vi "Smart_Oscilloscope.vi"() -> ()   [LabVIEW 2024]
uses:
  <vilib>/httpClient/POSTBuffer.vi
  <vilib>/httpClient/LabVIEWHTTPClient.lvlib
panel:
  in  "AI诊断":bool
  out "String":string
  in  "保存数据":bool
  in  "单次采集":bool
  in  "停止程序":bool
  in  "开始采集":bool
  in  "水平基准":dbl(knob) scale=0.0..10.0
  in  "垂直档位":dbl(knob) scale=0.0..10.0
  in  "采样率":dbl(knob) scale=0.0..10.0
  out "Waveform Graph":dynamicdata(graph)
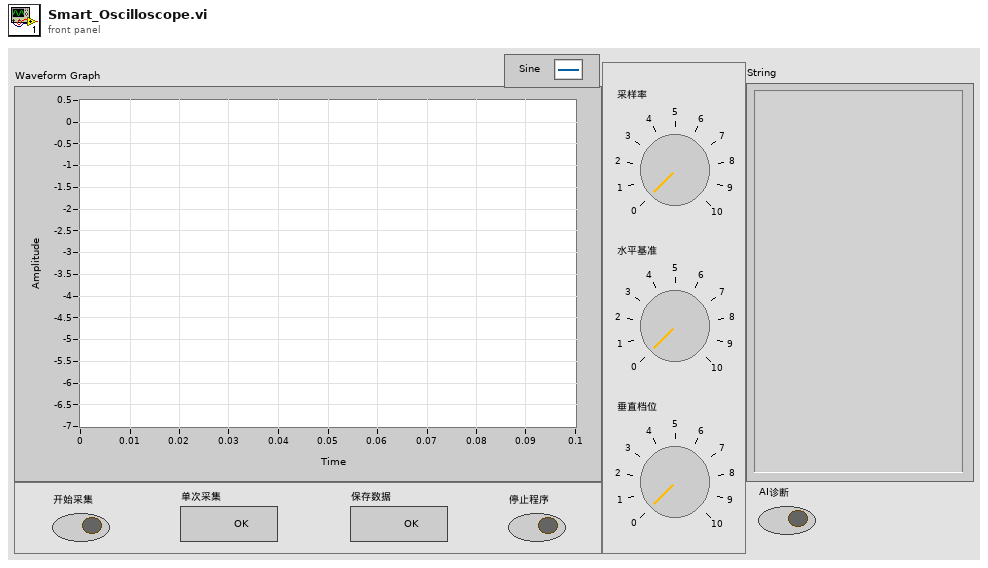
[diagram p1: front panel]
types:
  T1 = typedef "LabVIEWHTTPClient.lvlib/ClientHandle.ctl" = refnum<k1>
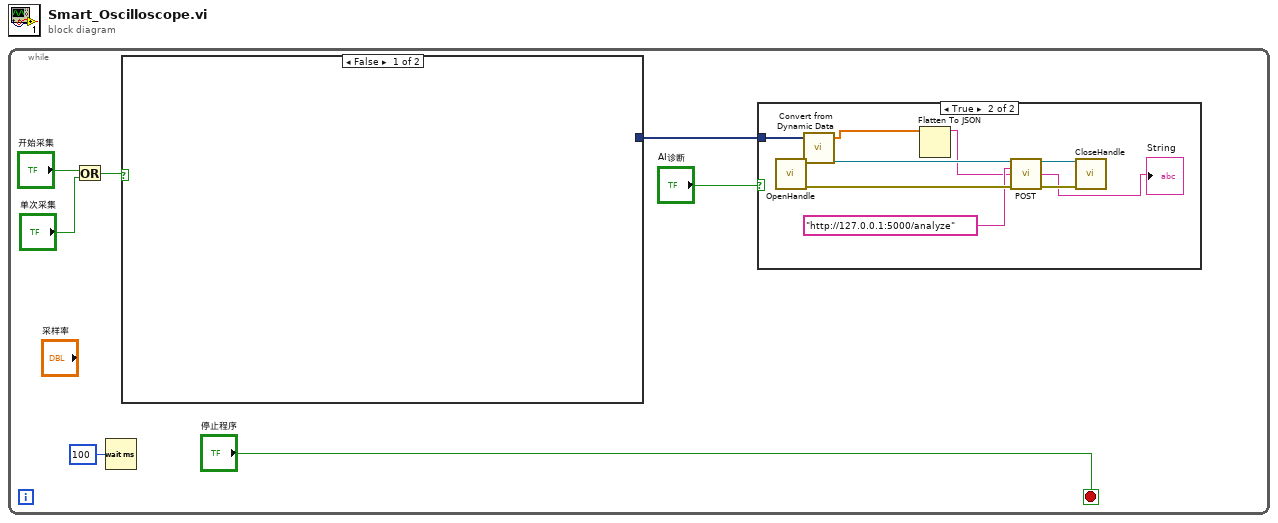
[diagram p0: block diagram]
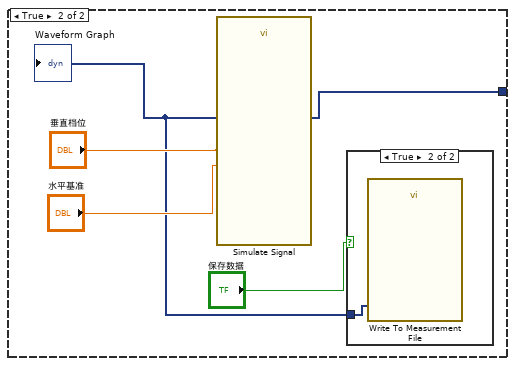
[diagram p3: hidden frame]
diagram:
  n1 = while {
    stop <- "停止程序" stop-if-true
    n2 = Or(x="开始采集", y="单次采集") -> (x .or. y?=w3:bool)
    n3 = Wait (ms)(milliseconds to wait=u32 100) -> ()  [unwired: 1 out]
    n4 = case shown="False" w3 {
      tunnel: [_ w17] -> w1
      frame False {
      }
      frame True {
        n5 = call "Simulate Signal"("Frequency"="水平基准", "Amplitude"="垂直档位") -> ("Sine"=w17:dynamicdata)  [unwired: 12 in, 1 out]
        "Waveform Graph" <- w17
        n6 = case shown="True" "保存数据" {
          tunnel: w17 -> [_ w21]
          frame False {
          }
          frame True {
            n7 = call "Write To Measurement File"("Signals"=w21) -> ()  [unwired: 16 in, 3 out]
          }
        }
      }
    }
    n8 = case shown="True" "AI诊断" {
      tunnel: w1 -> [_ w10]
      frame False {
      }
      frame True {
        n9 = call <vilib>:"OpenHandle.vi"() -> ("client handle out"=w13:T1, "error out"=w14:errorcluster)  [unwired: 14 in]
        n10 = call "Convert from Dynamic Data"("Dynamic Data Type"=w10) -> ("Array"=w9:dbl[])  [unwired: 3 in]
        n11 = Flatten To JSON(anything=w9) -> (JSON string=w8:string)  [unwired: 2 in, 1 out]
        n12 = call-poly <vilib>:"POST.vi"("client handle"=w13, "url"="http://127.0.0.1:5000/analyze", "buffer"=w8, "error in (no error)"=w14) -> ("client handle out"=w15:T1, "body"=→"String":string, "error out"=w16:errorcluster)  [unwired: 8 in, 1 out]
        n13 = call <vilib>:"CloseHandle.vi"("client handle"=w15, "error in (no error)"=w16) -> ()  [unwired: 13 in, 1 out]
      }
    }
  }
